vi "Write Short Name.vi"(8 "error in (no error)":errorcluster, 10 "Short Name":string, 11 "Generic Item in":refnum<class "Generic Item.lvclass">) -> (0 "error out":errorcluster, 3 "Generic Item out":refnum<class "Generic Item.lvclass">)   [LabVIEW 2015, in "Item Actor.lvlib" / "Generic Item.lvclass"]
uses:
  Generic Item.lvclass
  Generic Item.lvclass/Generic Item.ctl
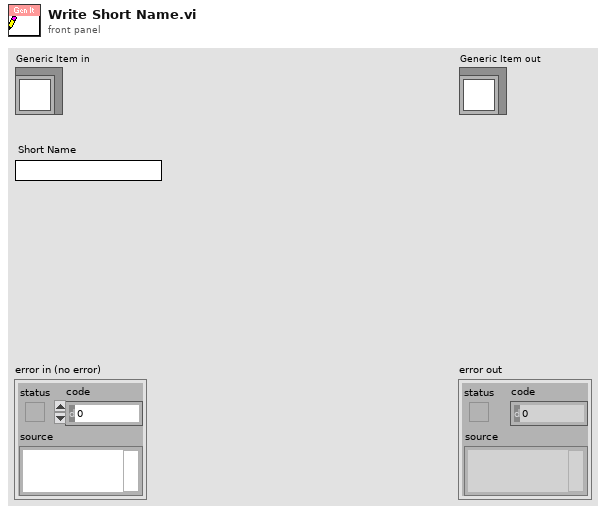
[diagram p1: front panel]
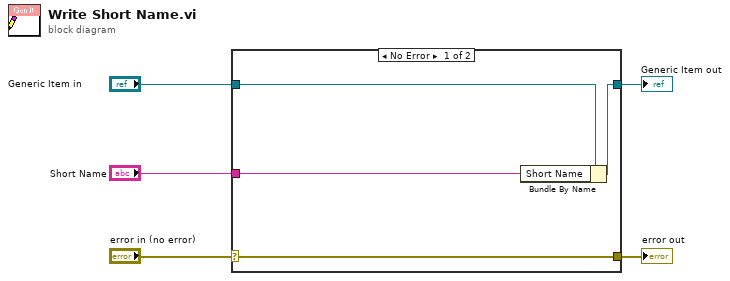
[diagram p0: block diagram]
diagram:
  n1 = case shown="No Error" "error in (no error)" {
    selector: "error in (no error)" -> [w9 w10]
    tunnel: [w9 w10] -> w4
    tunnel: [w7 w11] -> w2
    tunnel: "Generic Item in" -> [w8 w11]
    tunnel: "Short Name" -> [w6 _]
    frame No Error {
      n2 = Bundle By Name(cluster=w8, "Short Name"=w6) -> (w7:refnum<class "Generic Item.lvclass">)
    }
    frame Error {
    }
  }
  "error out" <- w4
  "Generic Item out" <- w2
